vi "Periodic Tasks.vi"(8 "error in":errorcluster) -> ()   [LabVIEW 2016]
doc: "This VI runs in parallel to other tasks. It can contain as many user-defined periodic loops as you need. These can carry out PID or other sorts of timed response."
uses:
  <vilib>/Platform/TimedLoop/XDataNode/timing_clust.ctl
  <vilib>/Platform/TimedLoop/XDataNode/nitl_modes.ctl
  <vilib>/Platform/TimedLoop/XDataNode/wakeup.ctl
  Robot Global Reference.vi
  <vilib>/platform/TimedLoop/XDataNode/XDataNode.xnode
  <vilib>/Platform/TimedLoop/XDataNode/XDNodeRunTimeDep.lvlib
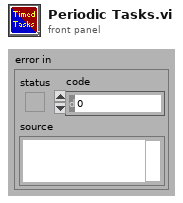
[diagram p1: front panel]
types:
  T1 = typedef "Joystick Reference.ctl" = cluster{"Driver Joystick":T2, "Operator Joystick":T2}
  T2 = typedef "WPI_JoystickDevRef.ctl" = cluster{"Device":T3}
  T3 = typedef "WPI_JoystickDeviceEnum.ctl" = enum16{"USB 0", "USB 1", "USB 2", "USB 3", "USB 4", "USB 5"}
  T4 = typedef "Drive Reference.ctl" = cluster{"RobotDriveDevRef":T5, "Drive PTO Solenoid":T10, "High Gear Solenoid":T10}
  T5 = typedef "WPI_RobotDriveDevRef.ctl" = cluster{"DevStatus":errorcluster, "Motors[]":T6[], "Square Inputs":bool, "Max Output":dbl}
  T6 = typedef "WPI_MotorControlDeviceRef.ctl" = cluster{"DeviceStatus":errorcluster, "Type":T7, "PWM":cluster{"PWM Channel":T8, "DeadBand":T9}, "CAN":cluster{"Device Number":u8, "SetOutput VI Ref":variant, "GetOutput VI Ref":variant, "Enable VI Ref":variant, "Disable VI Ref":variant, "Data":variant}, "Invert":bool}
  T7 = typedef "WPI_MotorControlType.ctl" = enum16{"PWM", "CAN"}
  T8 = typedef "FPGA_DIOPWMChannel.ctl" = enum8{"PWM 0", "PWM 1", "PWM 2", "PWM 3", "PWM 4", "PWM 5", "PWM 6", "PWM 7", "PWM 8", "PWM 9", "PWM MXP 0", "PWM MXP 1", "PWM MXP 2", "PWM MXP 3", "PWM MXP 4", "PWM MXP 5", "PWM MXP 6", "PWM MXP 7", "PWM MXP 8", "PWM MXP 9", "Invalid"}
  T9 = typedef "WPI_PWMDeadband.ctl" = cluster{"Name":string, "maxPositivePwm":i32, "minPositivePwm":i32, "centerPwm":i32, "maxNegativePwm":i32, "minNegativePwm":i32, "angularRange":u16}
  T10 = typedef "WPI_SolenoidDevRef.ctl" = cluster{"DevStatus":errorcluster, "Pneumatics Control Module":u8, "Forward Solenoid Channel":T11, "Reverse Solenoid Channel":T11}
  T11 = typedef "WPI_SolenoidChannel.ctl" = enum8{"Solenoid 0", "Solenoid 1", "Solenoid 2", "Solenoid 3", "Solenoid 4", "Solenoid 5", "Solenoid 6", "Solenoid 7", "Invalid"}
  T12 = typedef "Sensor Reference.ctl" = cluster{"LeftMotorEncoderRef":T13, "RightMotorEncoderRef":T13, "I2C Gyro":T17, "Left Shooter Wheel Encoder":T13, "Ultrasonic AIDeviceRef":T19}
  T13 = typedef "WPI_EncoderDevRef.ctl" = cluster{"DevStatus":errorcluster, "EncoderIndex":T14, "CounterIndex":T15, "DistancePerCount":dbl, "Decoding Type":T16}
  T14 = typedef "FPGA_EncoderIdx.ctl" = enum8{"Enc 0", "Enc 1", "Enc 2", "Enc 3", "Enc 4", "Enc 5", "Enc 6", "Enc 7", "Invalid"}
  T15 = typedef "FPGA_CounterCtrSystemIndex.ctl" = enum8{"Ctr 0", "Ctr 1", "Ctr 2", "Ctr 3", "Ctr 4", "Ctr 5", "Ctr 6", "Ctr 7", "Invalid"}
  T16 = typedef "WPI_EncoderType.ctl" = enum16{"1x", "2x", "4x"}
  T17 = typedef "WPI_I2CDevRef.ctl" = cluster{"DevStatus":errorcluster, "Device Address":u8, "Handle":i32, "I2C Bus":T18}
  T18 = typedef "i2c_bus.ctl" = enum16{"I2C On-Board", "I2C MXP", "Invalid"}
  T19 = typedef "WPI_AnalogChannelDevRef.ctl" = cluster{"DevStatus":errorcluster, "Analog Channel":T20}
  T20 = typedef "FPGA_AIChannel.ctl" = enum8{"AI 0", "AI 1", "AI 2", "AI 3", "AI MXP 0", "AI MXP 1", "AI MXP 2", "AI MXP 3", "Invalid"}
  T21 = typedef "Shoot Reference.ctl" = cluster{"Shooter Wheel Left":T6, "Shooter Wheel Right":T6, "Acquisition Conveyor Motor DevRef":T6, "Hopper Beater Bar Motor DevRef":T6}
  T22 = typedef "Gear Reference.ctl" = cluster{"Gear Ejection Cylinder":T10, "Door Ejection Cylinder":T10}
  T23 = typedef "Light Reference.ctl" = cluster{"SerialPortRef":T24}
  T24 = typedef "WPI_SerialPortRef.ctl" = cluster{"DevStatus":errorcluster, "Serial Port Name":refnum<visa-resource-name>}
  T25 = cluster{"Joystick Reference":T1, "Drive Reference":T4, "Sensor Reference":T12, "Shoot + Aquisition Reference":T21, "Gear Reference":T22, "Acquisition Conveyor Motor DevRef":T6, "Lights":T23}
  T26 = typedef "XDNodeRunTimeDep.lvlib/timing_clust.ctl" = cluster{"Expected End [f-1]":u64, "Actual End [f-1]":u64, "Finished Late? [f-1]":bool, "Expected End [i-1]":u64, "Actual End [i-1]":u64, "Finished Late? [i-1]":bool, "Expected Start [i]":u64, "Actual Start [i]":u64, "Expected Start [f]":u64, "Actual Start [f]":u64, "Source Name":string, "Structure Name":string, "Period":i64, "Deadline":i64, "Offset":i64, "Start":i64, "Priority":i32, "Timeout":i32, "Mode":T27, "Wakeup Reason":T28, "Error":errorcluster, "Source Type":string, "Secondary Source Type":string, "Global End Time":u64, "Global Start Time":u64, "Frame Duration":u64, "Iteration Duration":u64, "Assigned CPU":i32, "I/O Scan Engine Mode":u32}
  T27 = typedef "XDNodeRunTimeDep.lvlib/nitl_modes.ctl" = enum32{"No Change", "Process missed periods, maintain original phase", "Discard missed periods, maintain original phase", "Process missed periods, ignore original phase", "Discard missed periods, ignore original phase"}
  T28 = typedef "XDNodeRunTimeDep.lvlib/wakeup.ctl" = enum32{"Normal", "Aborted", "Asynchronous wakeup", "Timing source error", "Timed loop error", "Timeout"}
  T29 = typedef "Robot Values.ctl" = cluster{"Robot Drive":cluster{"Left Motor Power":dbl, "Right Motor Power":dbl, "Left Encoder Value":dbl, "Right Encoder Value":dbl, "High Gear?":bool, "PTO?":bool}, "Sensors":cluster{"Gyro Angle":u16, "Recalibrate Gyro":bool, "Reset Gyro":bool, "Ultrasonic":dbl}, "Shooter":cluster{"Prep Wheels":bool, "Shoot":bool, "Left Shooter Wheel Speed":dbl, "Wheels Moving":bool, "Shooter Prepped":bool, "Shooter RPS SP":dbl, "Shooting?":bool, "Left Shooter Wheel Power":dbl, "Right Shooter Wheel Power":dbl, "Acquisition Conveyor Power":dbl, "Hopper Beater Bar Power":dbl, "Filtered Left Shooter Speed":dbl, "Acquisition Motor Power":dbl, "Joystick Add":dbl, "D-Pad Add":dbl, "Shooter Use PID?":bool}, "Robot States":cluster{"Drive mode":string, "Alliance":T30, "Position":T31}, "Gear":cluster{"Ejection Active":bool}}
  T30 = typedef "WPI_DriverStationAllianceInfo.ctl" = enum16{"Red", "Blue", "Invalid"}
  T31 = typedef "WPI_DriverStationPositionInfo.ctl" = enum16{"1", "2", "3"}
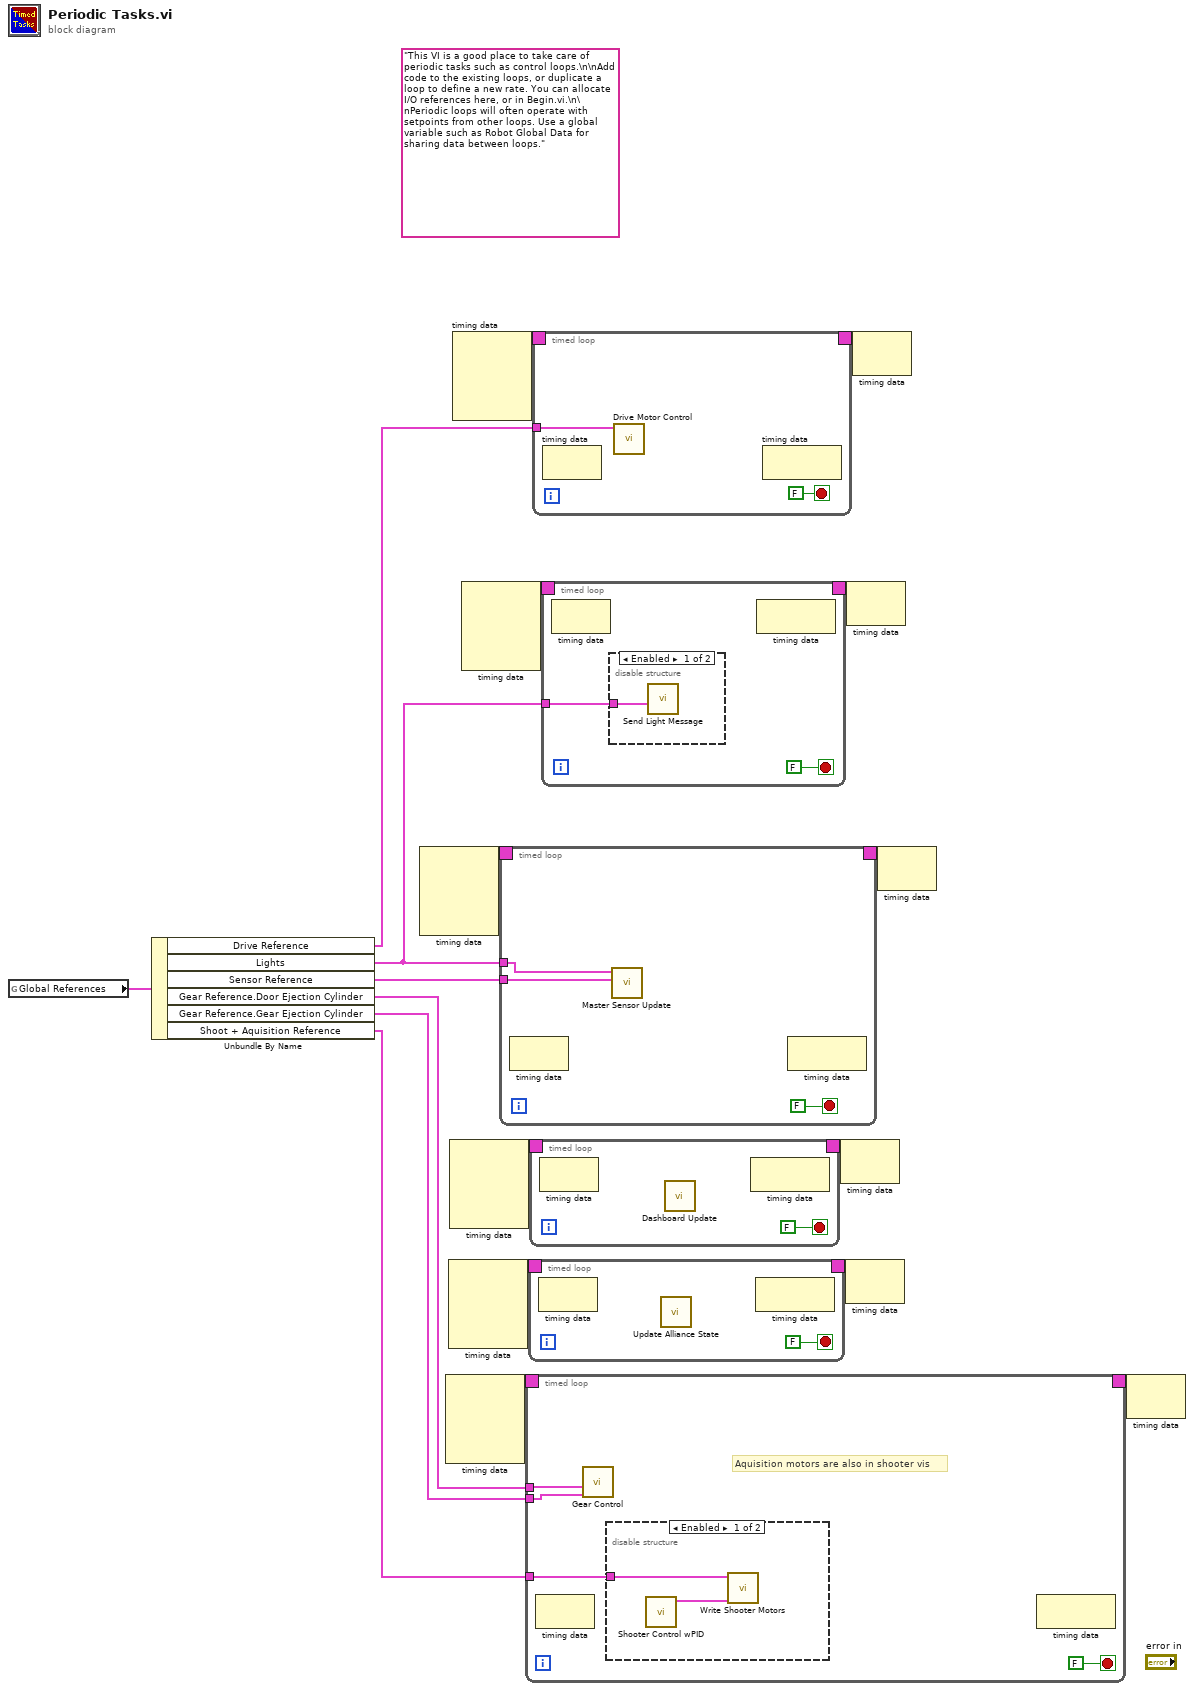
[diagram p0: block diagram]
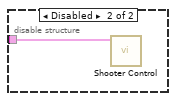
[diagram p3: hidden frame]
diagram:
  (unwired) "This VI is a good place to take care of periodic tasks such as control loops.\n\nAdd code to the existing loops, or duplicate a loop to define a new rate. You can allocate I/O references here, or in Begin.vi.\n\nPeriodic loops will often operate with setpoints from other loops. Use a global variable such as Robot Global Data for sharing data between loops."
  n1 = global read "Robot Global Reference.vi" "Global References"() -> (w19:T25)
  n2 = Unbundle By Name(w19) -> ("Drive Reference"=w11:T4, "Lights"=w1:T23, "Sensor Reference"=w14:T12, "Gear Reference.Door Ejection Cylinder"=w7:T10, "Gear Reference.Gear Ejection Cylinder"=w6:T10, "Shoot + Aquisition Reference"=w8:T21)
  n3 = node-c288() -> (w16:T26)  [unwired: 4 in]
  n4 = node-c288() -> (w13:T26)  [unwired: 4 in]
  n5 = node-c288() -> (w10:T26)  [unwired: 4 in]
  n6 = node-c288() -> (w3:T26)  [unwired: 4 in]
  n7 = node-c288() -> (w18:T26)  [unwired: 4 in]
  n8 = node-c288() -> (w5:T26)  [unwired: 4 in]
  n9 = timed-loop {
    timing: w16 -> [_]
    timing-out: [_] -> w15
    tunnel: w14 -> [w21]
    tunnel: w1 -> [w20]
    stop <- FALSE stop-if-true
    n10 = node-c288() -> ()  [unwired: 1 in, 1 out]
    n11 = call "Master Sensor Update.vi"("Sensor Reference Input"=w21, "Lights"=w20) -> ()  [unwired: 9 in, 1 out]
    n12 = node-c288() -> ()  [unwired: 1 in, 1 out]
  }
  n13 = timed-loop {
    timing: w13 -> [_]
    timing-out: [_] -> w12
    tunnel: w8 -> [w28]
    tunnel: w7 -> [w26]
    tunnel: w6 -> [w25]
    stop <- FALSE stop-if-true
    # "Aquisition motors are also in shooter vis"
    n14 = node-c288() -> ()  [unwired: 1 in, 1 out]
    n15 = call "Gear Control.vi"("Kicker SolenoidDevRefIn"=w25, "Gear Door SolenoidDevRefIn"=w26) -> ()  [unwired: 8 in, 2 out]
    n16 = disable-structure shown="Enabled" {
      disable-tunnel: w28 -> [w30 w31]
      frame Enabled {
        n17 = call "Shooter Control wPID.vi"() -> ("Robot Values Output"=w29:T29)  [unwired: 10 in]
        n18 = call "Write Shooter Motors.vi"("Robot Values Input"=w29, "Shoot Reference In"=w30) -> ()  [unwired: 9 in, 1 out]
      }
      frame Disabled {
        n19 = call "Shooter Control.vi"("Shoot Reference In"=w31) -> ()  [unwired: 10 in, 1 out]
      }
    }
    n20 = node-c288() -> ()  [unwired: 1 in, 1 out]
  }
  n21 = timed-loop {
    timing: w10 -> [_]
    timing-out: [_] -> w9
    stop <- FALSE stop-if-true
    n22 = node-c288() -> ()  [unwired: 1 in, 1 out]
    n23 = call "Update Alliance State.vi"() -> ()  [unwired: 12 in]
    n24 = node-c288() -> ()  [unwired: 1 in, 1 out]
  }
  n25 = timed-loop {
    timing: w3 -> [_]
    timing-out: [_] -> w2
    stop <- FALSE stop-if-true
    n26 = node-c288() -> ()  [unwired: 1 in, 1 out]
    n27 = call "Dashboard Update.vi"() -> ()  [unwired: 12 in]
    n28 = node-c288() -> ()  [unwired: 1 in, 1 out]
  }
  n29 = timed-loop {
    timing: w18 -> [_]
    timing-out: [_] -> w17
    tunnel: w11 -> [w40]
    stop <- FALSE stop-if-true
    n30 = node-c288() -> ()  [unwired: 1 in, 1 out]
    n31 = call "Drive Motor Control.vi"("Drive Reference In"=w40) -> ()  [unwired: 10 in, 1 out]
    n32 = node-c288() -> ()  [unwired: 1 in, 1 out]
  }
  n33 = timed-loop {
    timing: w5 -> [_]
    timing-out: [_] -> w4
    tunnel: w1 -> [w44]
    stop <- FALSE stop-if-true
    n34 = node-c288() -> ()  [unwired: 1 in, 1 out]
    n35 = disable-structure shown="Enabled" {
      disable-tunnel: w44 -> [w46 _]
      frame Enabled {
        n36 = call "Send Light Message.vi"("Lights"=w46) -> ()  [unwired: 10 in, 1 out]
      }
      frame Disabled {
      }
    }
    n37 = node-c288() -> ()  [unwired: 1 in, 1 out]
  }
  n38 = node-c288(w2) -> ()  [unwired: 1 out]
  n39 = node-c288(w9) -> ()  [unwired: 1 out]
  n40 = node-c288(w4) -> ()  [unwired: 1 out]
  n41 = node-c288(w17) -> ()  [unwired: 1 out]
  n42 = node-c288(w15) -> ()  [unwired: 1 out]
  n43 = node-c288(w12) -> ()  [unwired: 1 out]
